vi "Read Append Numeric.vi"(11 "StringIncrementAlgorithm in":refnum<class "StringIncrementAlgorithm.lvclass">) -> (2 "Append Numeric":u32, 3 "StringIncrementAlgorithm out":refnum<class "StringIncrementAlgorithm.lvclass">)   [LabVIEW 2014, in "UniqueName.lvlib" / "StringIncrementAlgorithm.lvclass"]
uses:
  StringIncrementAlgorithm.lvclass
  StringIncrementAlgorithm.lvclass/StringIncrementAlgorithm.ctl
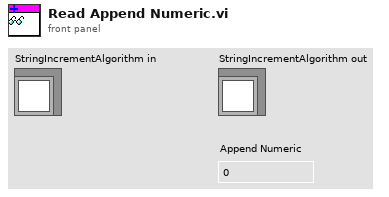
[diagram p1: front panel]
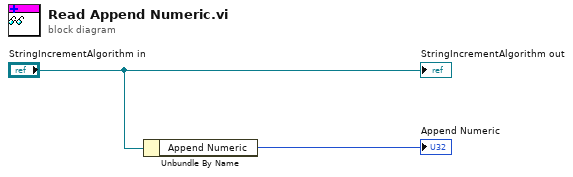
[diagram p0: block diagram]
diagram:
  n1 = Unbundle By Name("StringIncrementAlgorithm in") -> ("Append Numeric"=→"Append Numeric":u32)
  "StringIncrementAlgorithm out" <- "StringIncrementAlgorithm in"
